vi "Update.vi"(8 "error in (no error)":errorcluster, 10 "username":string, 11 "[Data] Recent User in":refnum<class "[User] Recent Login.lvclass">) -> (0 "error out":errorcluster, 3 "[Data] Recent User out":refnum<class "[User] Recent Login.lvclass">)   [LabVIEW 2020, in "[User] Recent Login.lvclass"]
uses:
  [User] Recent Login.lvclass
  [User] Recent Login.lvclass/[User] Recent Login.ctl
  324536a1-1b90-4293-b119-883fe3d1fe02.vi
  <vilib>/Comparison/Equal/Equal Functor/Equal Functor.lvclass
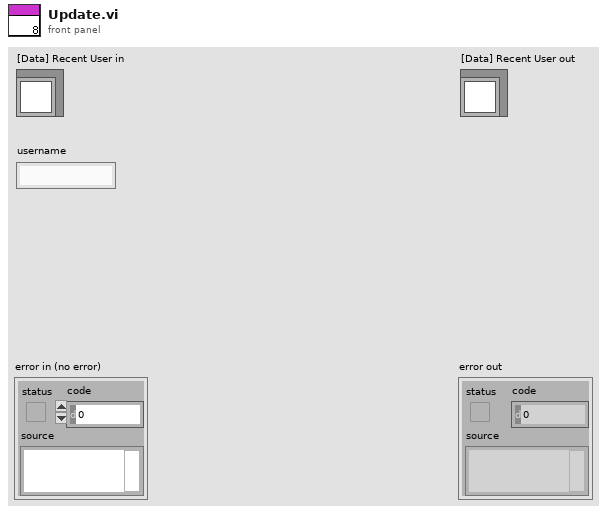
[diagram p1: front panel]
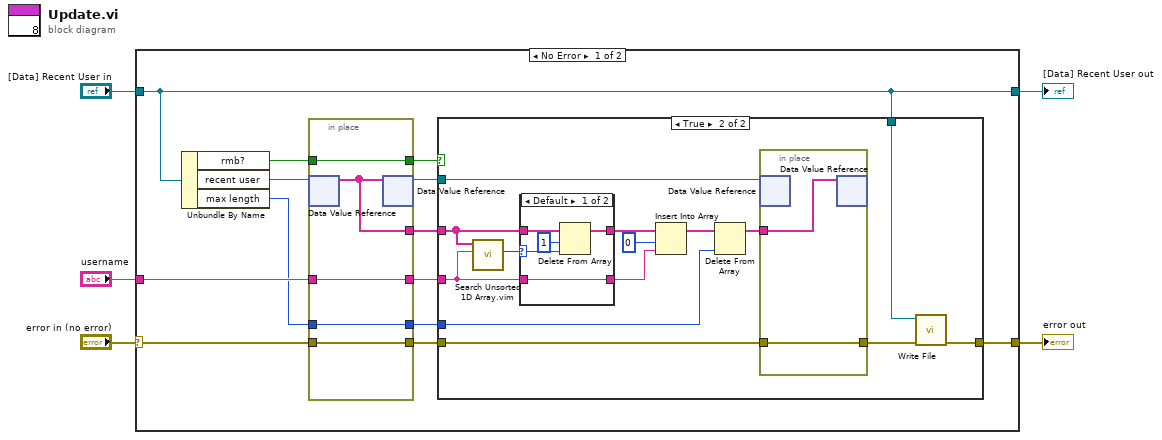
[diagram p0: block diagram]
diagram:
  n1 = case shown="No Error" "error in (no error)" {
    selector: "error in (no error)" -> [w16 w49]
    tunnel: [w8 w49] -> w4
    tunnel: [w9 w48] -> w2
    tunnel: "[Data] Recent User in" -> [w9 w48]
    tunnel: "username" -> [w17 _]
    frame No Error {
      n2 = Unbundle By Name(w9) -> ("rmb?"=w7:bool, "recent user"=w18:refnum<data-value>, "max length"=w12:u8)
      n3 = in-place {
        in-place-border: w17 -> [w46]
        in-place-border: w16 -> [w47]
        in-place-border: [w47] -> w10
        in-place-border: [w46] -> w14
        in-place-border: [w44] -> w15
        in-place-border: w12 -> [w45]
        in-place-border: [w45] -> w11
        in-place-border: w7 -> [w43]
        in-place-border: [w43] -> w6
        n4 = in-place-dvr #1(w18) -> (w44:string[])  [unwired: 1 out]
        n5 = in-place-dvr #1(w44) -> (w13:refnum<data-value>)  [unwired: 1 out]
      }
      n6 = case shown="True" w6 {
        tunnel: w15 -> [_ w32]
        tunnel: w14 -> [_ w31]
        tunnel: w13 -> [_ w25]
        tunnel: w11 -> [_ w26]
        tunnel: w10 -> [w19 w23]
        tunnel: [w19 w20] -> w8
        tunnel: w9 -> [_ w21]
        frame False {
        }
        frame True {
          n7 = call "Search Unsorted 1D Array.vim"("element"=w31, "unsorted 1D array"=w32) -> ("index of element"=w33:i32)  [unwired: 9 in]
          n8 = case shown="Default" w33 {
            selector: w33 -> [w37 _]
            tunnel: w32 -> [w39 w42]
            tunnel: w31 -> [w40 w41]
            tunnel: [w38 w42] -> w30
            tunnel: [w40 w41] -> w29
            frame Default {
              n9 = Delete From Array(array=w39, length=1, index=w37) -> (array with subset deleted=w38:string[])  [unwired: 1 out]
            }
            frame -1 {
            }
          }
          n10 = Insert Into Array(array=w30, index=0, new element=w29) -> (w27:string[])
          n11 = Delete From Array(array=w27, index=w26) -> (array with subset deleted=w24:string[])  [unwired: 1 in, 1 out]
          n12 = in-place {
            in-place-border: w23 -> [w35]
            in-place-border: [w35] -> w22
            in-place-border: w24 -> [w34]
            n13 = in-place-dvr #2(w25) -> ()  [unwired: 2 out]
            n14 = in-place-dvr #2(w34) -> ()  [unwired: 2 out]
          }
          n15 = call "Write File.vi"("error in (no error)"=w22, "[Data] Recent User in"=w21) -> ("error out"=w20:errorcluster)  [unwired: 8 in, 1 out]
        }
      }
    }
    frame Error {
    }
  }
  "error out" <- w4
  "[Data] Recent User out" <- w2
